vi "Update Value.vi"(8 "error in (no error)":errorcluster, 10 "Type Value":refnum<class "Type.lvclass">, 11 "ColumnPanel in":refnum<class "ColumnPanel.lvclass">) -> (0 "error out":errorcluster, 3 "ColumnPanel out":refnum<class "ColumnPanel.lvclass">)   [LabVIEW 2020, in "Conditum-Tools.lvlib" / "ColumnPanel.lvclass"]
uses:
  ColumnPanel.lvclass
  ColumnPanel.lvclass/ColumnPanel.ctl
  Conditum/Columns/Type/Type.lvclass
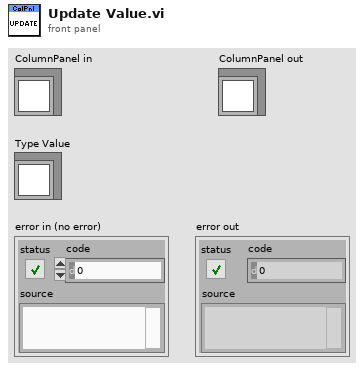
[diagram p1: front panel]
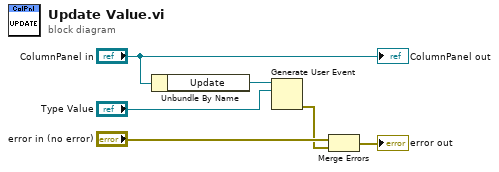
[diagram p0: block diagram]
diagram:
  n1 = Unbundle By Name("ColumnPanel in") -> ("Update"=w4:refnum<user-event>)
  n2 = Generate User Event(user event=w4, event data cluster="Type Value") -> (error out=w2:errorcluster)  [unwired: 2 in, 1 out]
  n3 = Merge Errors("error in (no error)", w2) -> (→"error out":errorcluster)
  "ColumnPanel out" <- "ColumnPanel in"
